vi "SCCSup Merge 2 Errors.vi"(12 "Error IO 1":errorcluster, 14 "Error IO 2":errorcluster) -> (2 "Error IO out":errorcluster)   [LabVIEW 2017]
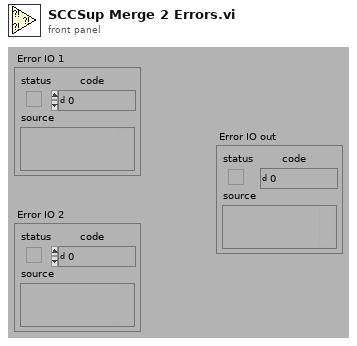
[diagram p1: front panel]
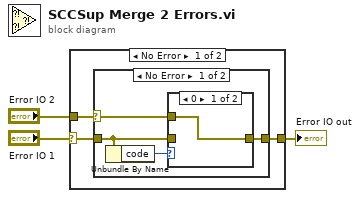
[diagram p0: block diagram]
diagram:
  n1 = case shown="No Error" "Error IO 1" {
    selector: "Error IO 1" -> [w4 w14]
    tunnel: [w5 w14] -> w1
    tunnel: "Error IO 2" -> [w6 _]
    frame No Error {
      n2 = case shown="No Error" w6 {
        selector: w6 -> [w8 w13]
        tunnel: [w9 w13] -> w5
        tunnel: w4 -> [w7 _]
        frame No Error {
          n3 = Unbundle By Name(w7) -> ("code"=w10:i32)
          n4 = case shown="0" w10 {
            tunnel: [w11 w12] -> w9
            tunnel: w8 -> [w11 _]
            tunnel: w7 -> [_ w12]
            frame 0 {
            }
            frame Default {
            }
          }
        }
        frame Error {
        }
      }
    }
    frame Error {
    }
  }
  "Error IO out" <- w1
